vi "Start Output Panel.vi"(7 "Project In":refnum<class "Project.lvclass">, 8 "error in (no error)":errorcluster, 10 "Panel Hostl Refnum":refnum<vi>, 11 "CallEXEStep in":refnum<class "CallEXEStep.lvclass">) -> (0 "error out":errorcluster, 2 "Panel VI Refnum":refnum<vi>, 3 "CallEXEStep out":refnum<class "CallEXEStep.lvclass">)   [LabVIEW 2015, in "CallEXEStep.lvclass"]
uses:
  CallEXEStep.lvclass
  Step.lvclass
  Project.lvclass
  OutputUI/Output Panel.vi
  OutputUI.lvclass
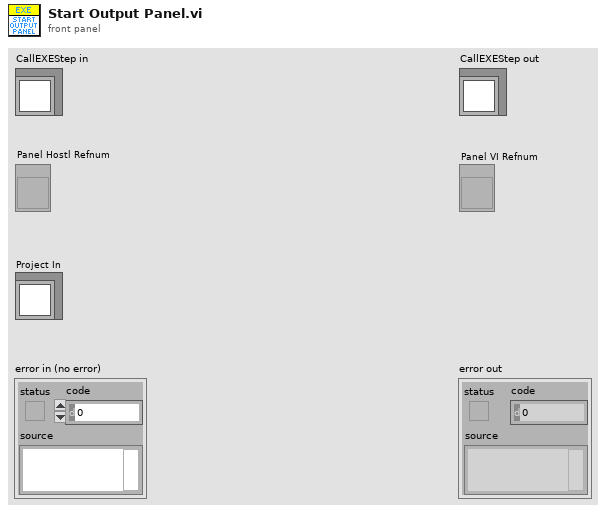
[diagram p1: front panel]
types:
  T1 = enum32{"Invalid", "Standard", "Closed", "Hidden", "Minimized", "Maximized"}
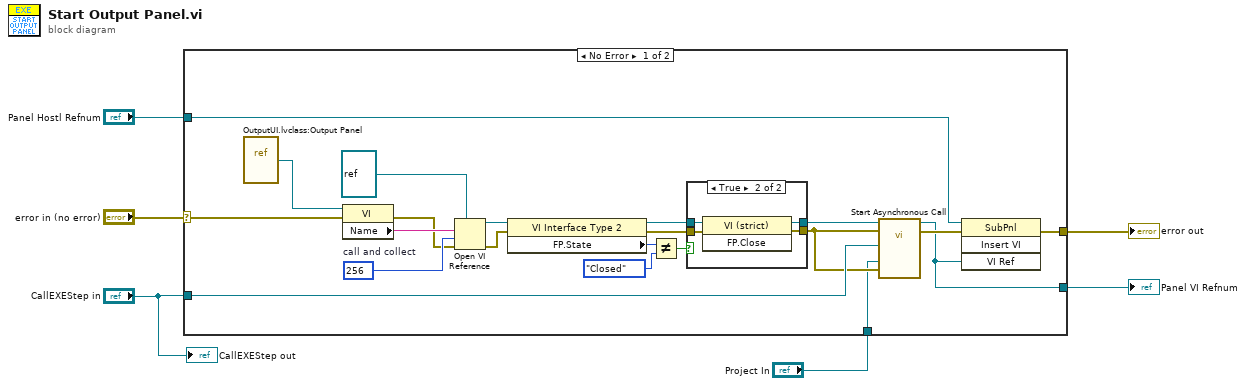
[diagram p0: block diagram]
diagram:
  n1 = case shown="No Error" "error in (no error)" {
    selector: "error in (no error)" -> [w27 w34]
    tunnel: [w26 w34] -> w3
    tunnel: "CallEXEStep in" -> [w25 _]
    tunnel: "Panel Hostl Refnum" -> [w9 _]
    tunnel: [w8 _] -> w2
    tunnel: "Project In" -> [w7 _]
    frame No Error {
      w21 = 256  # call and collect
      n2 = vi-ref "OutputUI.lvclass:Output Panel.vi"() -> (w24:refnum<vi>)
      n3 = property class="VI"(reference=w24, error in=w27) -> (error out=w19:errorcluster, "Name"=w22:string)  [unwired: 1 out]
      n4 = Open VI Reference(type specifier VI Refnum (for type only)=refnum<vi> refnum, vi path=w22, options=w21, error in (no error)=w19) -> (vi reference=w13:refnum<vi>, error out=w12:errorcluster)  [unwired: 2 in]
      n5 = property class="VI Interface Type 2"(reference=w13, error in=w12) -> (reference out=w17:refnum<vi>, error out=w18:errorcluster, "FP.State"=w14:T1)
      n6 = Not Equal?(x=w14, y=T1."Closed" ("Front Panel Window:State")) -> (x != y?=w16:bool)
      n7 = case shown="True" w16 {
        tunnel: w17 -> [w29 w33]
        tunnel: w18 -> [w28 w32]
        tunnel: [w29 w31] -> w11
        tunnel: [w28 w30] -> w10
        frame False {
        }
        frame True {
          n8 = invoke class="VI (strict)" method="FP.Close"(reference=w33, error in=w32) -> (reference out=w31:refnum<vi>, error out=w30:errorcluster)  [unwired: 1 in, 1 out]
        }
      }
      n9 = call-by-ref "Start Asynchronous Call"(reference=w11, error in=w10, 8:"error in (no error)"=w10, "Project In"=w7, "Step in"=w25) -> (reference out=w8:refnum<vi>, error out=w20:errorcluster)  [unwired: 7 in, 2 out]
      n10 = invoke class="SubPnl" method="Insert VI"(reference=w9, error in=w20, "VI Ref"=w8) -> (error out=w26:errorcluster)  [unwired: 1 in, 3 out]
    }
    frame Error {
    }
  }
  "error out" <- w3
  "Panel VI Refnum" <- w2
  "CallEXEStep out" <- "CallEXEStep in"
